vi "InitConnection.vi"(8 "error in (no error)":errorcluster, 11 "Sync Box in":refnum<class "Sync Box.lvclass">) -> (0 "error out":errorcluster, 3 "Sync Box out":refnum<class "Sync Box.lvclass">)   [LabVIEW 2018, in "Sync Box.lvclass"]
uses:
  Sync Box.lvclass
  Trigger/Trigger.lvclass
  Server/Server.lvclass
  StateMachine/State Machine.lvclass
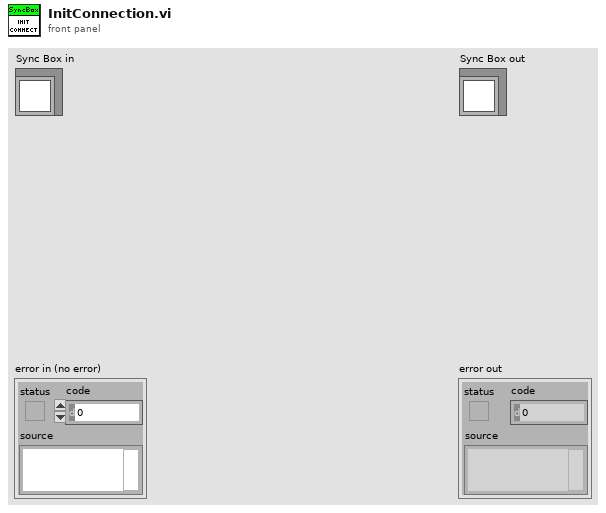
[diagram p1: front panel]
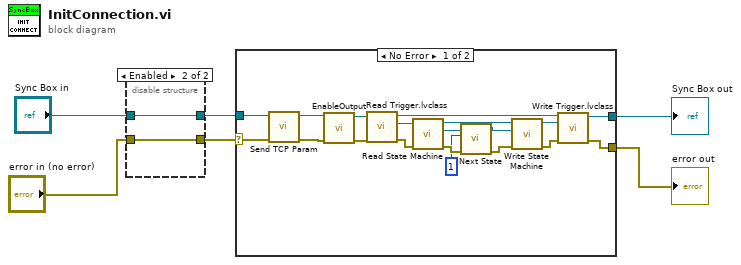
[diagram p0: block diagram]
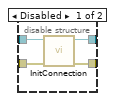
[diagram p2: hidden frame]
diagram:
  n1 = disable-structure shown="Enabled" {
    disable-tunnel: "error in (no error)" -> [w10 w11]
    disable-tunnel: "Sync Box in" -> [w9 w12]
    disable-tunnel: [w8 w12] -> w4
    disable-tunnel: [w7 w11] -> w3
    frame Disabled {
      n2 = call-parent "InitConnection.vi"("error in (no error)"=w10, "Server in"=w9) -> ("error out"=w7:errorcluster, "Server out"=w8:refnum<class "Sync Box.lvclass">)  [unwired: 8 in]
    }
    frame Enabled {
    }
  }
  n3 = case shown="No Error" w3 {
    selector: w3 -> [w14 w32]
    tunnel: w4 -> [w16 w33]
    tunnel: [w18 w32] -> w2
    tunnel: [w17 w33] -> w1
    frame No Error {
      n4 = call-dynamic "Send TCP Param.vi"("error in (no error)"=w14, "Server in"=w16) -> ("error out"=w13:errorcluster, "Server out"=w15:refnum<class "Sync Box.lvclass">)  [unwired: 8 in]
      n5 = call-dynamic "EnableOutput.vi"("error in (no error)"=w13, "Sync Box in"=w15) -> ("error out"=w26:errorcluster, "Sync Box out"=w31:refnum<class "Sync Box.lvclass">)  [unwired: 8 in]
      n6 = call-dynamic "Read Trigger.lvclass.vi"("error in (no error)"=w26, "Sync Box in"=w31) -> ("error out"=w25:errorcluster, "Trigger.lvclass"=w29:refnum<class "Trigger.lvclass">, "Sync Box out"=w30:refnum<class "Sync Box.lvclass">)  [unwired: 7 in]
      n7 = call-dynamic "Read State Machine.vi"("error in (no error)"=w25, "Device in"=w29) -> ("error out"=w24:errorcluster, "State Machine.lvclass"=w21:refnum<class "State Machine.lvclass">, "Device out"=w28:refnum<class "Trigger.lvclass">)  [unwired: 7 in]
      n8 = call "Next State.vi"("error in (no error)"=w24, "New_State"=u32 1, "State Machine in"=w21) -> ("error out"=w23:errorcluster, "State Machine out"=w20:refnum<class "State Machine.lvclass">)  [unwired: 7 in]
      n9 = call-dynamic "Write State Machine.vi"("error in (no error)"=w23, "State Machine.lvclass"=w20, "Device in"=w28) -> ("error out"=w22:errorcluster, "Device out"=w27:refnum<class "Trigger.lvclass">)  [unwired: 7 in]
      n10 = call-dynamic "Write Trigger.lvclass.vi"("error in (no error)"=w22, "Trigger.lvclass"=w27, "Sync Box in"=w30) -> ("error out"=w18:errorcluster, "Sync Box out"=w17:refnum<class "Sync Box.lvclass">)  [unwired: 7 in]
    }
    frame Error {
    }
  }
  "error out" <- w2
  "Sync Box out" <- w1
